vi "S2DS_WCFromFile.vi"(4 "Ramp Y to zero?":bool, 6 "Ramp X to zero?":bool, 7 "Scan parameters in":T1 {"Y data taking" items=["in both direction", "in up direction only", "in down direction only"]; "X data taking" items=["in both direction", "in up direction only", "in down direction only"]}, 8 "error in (no error)":errorcluster, 10 "WC read from file info (in)":T2, 11 "WC info list in":T3) -> (0 "error out":errorcluster, 1 "Index":i32, 2 "WC read from file info (out)":T2, 3 "WC info list out":T3, 5 "File over?":bool)   [LabVIEW 2025]
uses:
  TYPE DEFS/S2DS_WC info.ctl
  TYPE DEFS/S2DS_Single WC info.ctl
  TYPE DEFS/S2DS_WCFromFileInfo.ctl
  TYPE DEFS/S2DS_Sweep Info.ctl
  <vilib>/Utility/file.llb/Read Delimited Spreadsheet (DBL).vi
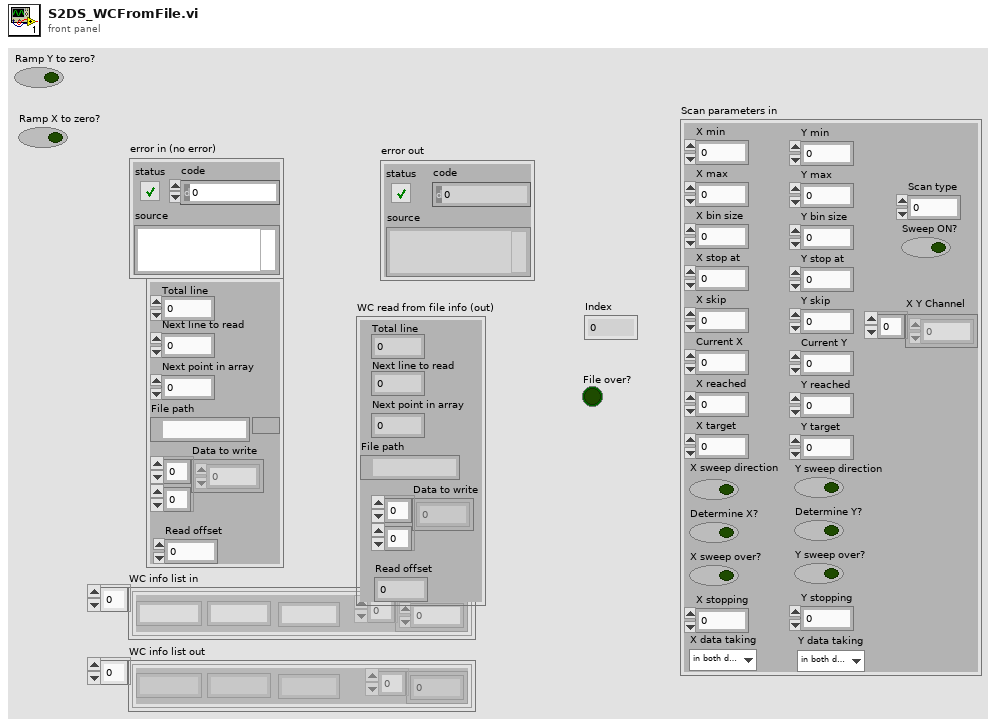
[diagram p1: front panel]
types:
  T1 = typedef "S2DS_Sweep Info.ctl" = cluster{"X min":ext, "X max":dbl, "Y min":dbl, "Y max":dbl, "X bin size":dbl, "Y bin size":dbl, "X stop at":dbl, "Y stop at":dbl, "X skip":u64, "Y skip":u64, "Current X":dbl, "Current Y":dbl, "X reached":i32, "Y reached":i32, "X target":dbl, "Y target":dbl, "Sweep ON?":bool, "X sweep direction":bool, "Y sweep direction":bool, "Determine X?":bool, "Determine Y?":bool, "X sweep over?":bool, "Y sweep over?":bool, "Scan type":i32, "X stopping":i32, "Y stopping":i32, "X Y Channel":u16[], "X data taking":u16, "Y data taking":u16}
  T2 = typedef "S2DS_WCFromFileInfo.ctl" = cluster{"Next line to read":i32, "Next point in array":i32, "File path":path, "Data to write":dbl[][], "Read offset":i32, "Total line":i32}
  T3 = typedef "S2DS_WC info.ctl" = T4[]
  T4 = typedef "S2DS_Single WC info.ctl" = cluster{"Instrument identifier":string, "Write channel parameters":dbl[], "Name":string, "Unit":string}
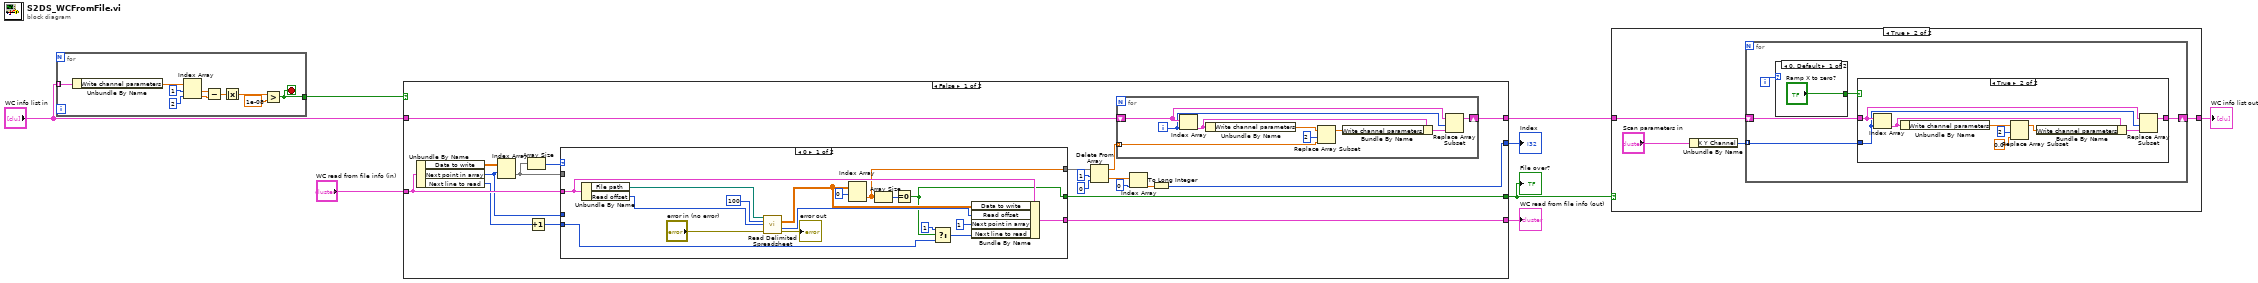
[diagram p0: block diagram]
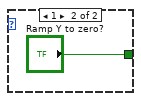
[diagram p4: hidden frame]
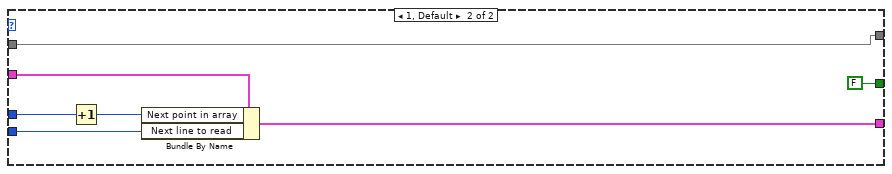
[diagram p5: hidden frame]
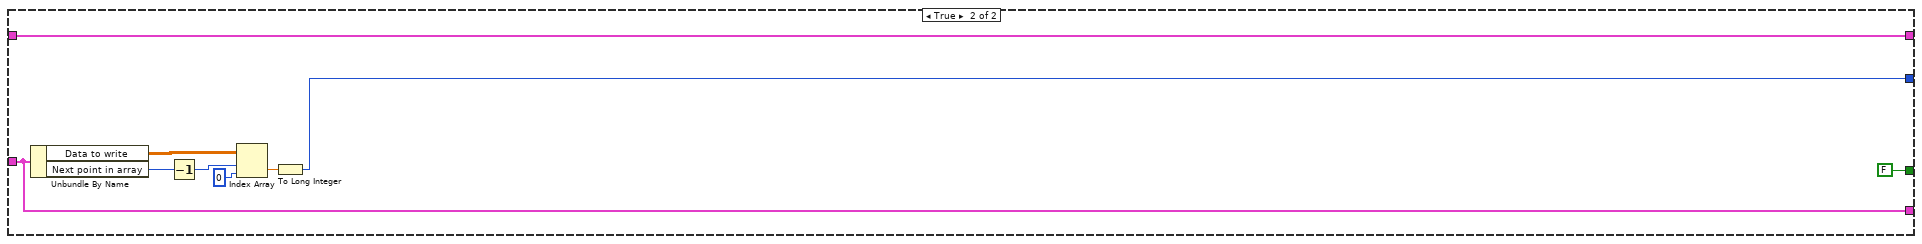
[diagram p6: hidden frame]
diagram:
  n1 = for {
    tunnel: "WC info list in" -> [w18] mode=indexing
    tunnel: [w9] -> w4
    stop <- w9 stop-if-true
    n2 = Unbundle By Name(w18) -> ("Write channel parameters"=w17:dbl[])
    n3 = Index Array(array=w17, index #1=1 ("index"), index #2=2 ("index")) -> (element #1=w14:dbl, element #2=w13:dbl)
    n4 = Subtract(x=w14, y=w13) -> (x-y=w12:dbl)
    n5 = Absolute Value(x=w12) -> (abs(x)=w11:dbl)
    n6 = Greater?(x=w11, y=1e-08) -> (0:w9:bool)
  }
  n7 = case shown="False" w4 {
    tunnel: "WC read from file info (in)" -> [w36 w77]
    tunnel: [w31 w79] -> w2
    tunnel: [w27 w71] -> w7
    tunnel: [w26 FALSE] -> w3
    tunnel: [w25 w77] -> w6
    tunnel: "WC info list in" -> [w19 w79]
    frame False {
      n8 = Unbundle By Name(w36) -> ("Data to write"=w24:dbl[][], "Next point in array"=w22:i32, "Next line to read"=w21:i32)
      n9 = Index Array(array=w24, index (row)=w22) -> (element=w23:dbl[])  [unwired: 1 in]
      n10 = Array Size(array=w23) -> (size(s)=w37:i32)
      n11 = Increment(x=w21) -> (x+1=w20:i32)
      n12 = case shown="0" w37 {
        tunnel: [w61 w68] -> w30
        tunnel: w23 -> [_ w68]
        tunnel: w36 -> [w63 w70]
        tunnel: [w62 w69] -> w25
        tunnel: [w50 FALSE] -> w26
        tunnel: w22 -> [_ w66]
        tunnel: w20 -> [w47 w64]
        frame 0 {
          n13 = Unbundle By Name(w63) -> ("File path"=w59:path, "Read offset"=w58:i32)
          n14 = call-poly <vilib>:"Read Delimited Spreadsheet.vi"("file path (dialog if empty)"=w59, "number of rows (all:-1)"=100, "start of read offset (chars.:0)"=w58, "error in (no error)"="error in (no error)") -> ("all rows"=w53:dbl[][], "mark after read (chars.)"=w57:i32, "error out"=→"error out":errorcluster)  [unwired: 6 in, 3 out]
          n15 = Index Array(array=w53, index (row)=0) -> (element=w61:dbl[])  [unwired: 1 in]
          n16 = Array Size(array=w61) -> (size(s)=w54:i32)
          n17 = Equal To 0?(x=w54) -> (x = 0?=w50:bool)
          n18 = Select(t=1, s=w50, f=w47) -> (s? t:f=w49:i32)
          n19 = Bundle By Name(cluster=w63, "Data to write"=w53, "Read offset"=w57, "Next point in array"=1, "Next line to read"=w49) -> (w62:T2)
        }
        frame 1, Default {
          n20 = Increment(x=w66) -> (x+1=w65:i32)
          n21 = Bundle By Name(cluster=w70, "Next point in array"=w65, "Next line to read"=w64) -> (w69:T2)
        }
      }
      n22 = Delete From Array(array=w30, length=1, index=0) -> (deleted portion=w34:dbl[], array with subset deleted=w35:dbl[])
      n23 = for {
        tunnel: w35 -> [w45] mode=indexing
        shift-right: [w40] -> w31
        shift-left: w19 -> [w43]
        i -> [w42]
        n24 = Index Array(array=w43, index=w42) -> (element=w39:T4)
        n25 = Unbundle By Name(w39) -> ("Write channel parameters"=w38:dbl[])
        n26 = Replace Array Subset(array=w38, new element=w45, index=2) -> (w44:dbl[])
        n27 = Bundle By Name(cluster=w39, "Write channel parameters"=w44) -> (w41:T4)
        n28 = Replace Array Subset(array=w43, new element=w41, index=w42) -> (w40:T3)
      }
      n29 = Index Array(array=w34, index=0) -> (element=w28:dbl)
      n30 = To Long Integer(number=w28) -> (32bit integer=w27:i32)
    }
    frame True {
      n31 = Unbundle By Name(w77) -> ("Data to write"=w76:dbl[][], "Next point in array"=w75:i32)
      n32 = Decrement(x=w75) -> (x-1=w74:i32)
      n33 = Index Array(array=w76, index (row)=w74, index (col)=0 ("disabled index (col)")) -> (element=w72:dbl)
      n34 = To Long Integer(number=w72) -> (32bit integer=w71:i32)
    }
  }
  "Index" <- w7
  "File over?" <- w3
  "WC read from file info (out)" <- w6
  n35 = case shown="True" w3 {
    tunnel: w2 -> [w80 w82]
    tunnel: [w80 w81] -> w1
    frame False {
    }
    frame True {
      n36 = Unbundle By Name("Scan parameters in") -> ("X Y Channel"=w83:u16[])
      n37 = for {
        tunnel: w83 -> [w85] mode=indexing
        shift-right: [w86] -> w81
        shift-left: w82 -> [w87]
        i -> [w89]
        n38 = case shown="0, Default" w89 {
          tunnel: ["Ramp X to zero?" "Ramp Y to zero?"] -> w88
          frame 0, Default {
          }
          frame 1 {
          }
        }
        n39 = case shown="True" w88 {
          tunnel: w87 -> [w90 w94]
          tunnel: [w90 w93] -> w86
          tunnel: w85 -> [_ w92]
          frame False {
          }
          frame True {
            n40 = Index Array(array=w94, index=w92) -> (element=w96:T4)
            n41 = Unbundle By Name(w96) -> ("Write channel parameters"=w97:dbl[])
            n42 = Replace Array Subset(array=w97, new element=0.0 ("new element/subarray"), index=2) -> (w98:dbl[])
            n43 = Bundle By Name(cluster=w96, "Write channel parameters"=w98) -> (w95:T4)
            n44 = Replace Array Subset(array=w94, new element=w95, index=w92) -> (w93:T3)
          }
        }
      }
    }
  }
  "WC info list out" <- w1
